vi "SEA_9811_Create_Send_Channels.vi"(8 "error in (no error)":errorcluster, 11 "Item Ref in":T1 format="%.0x") -> (0 "error out":errorcluster, 3 "Item Ref out":T1 format="%.0x")   [LabVIEW 2015, in "AIT 429 System Explorer.lvlib"]
uses:
  AIT 429 System Explorer.lvlib
  <vilib>/NI Veristand/Custom Device API/Custom Device Item Ref.ctl
  <vilib>/NI Veristand/Custom Device API/Custom Device Channel.ctl
  <vilib>/NI Veristand/Custom Device API/Custom Device Channel Type.ctl
  Shared/Controls and Global/Global.vi
  <vilib>/NI Veristand/Custom Device API/Custom Device API.lvlib
  Shared/AIT 429 Shared.lvlib
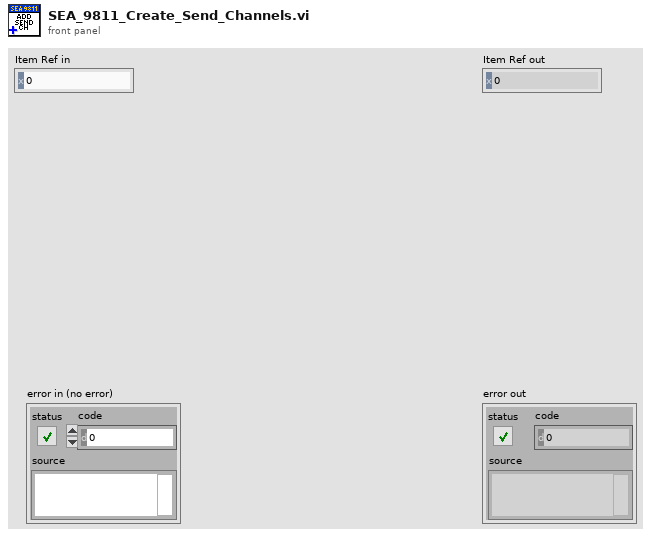
[diagram p1: front panel]
types:
  T1 = typedef "Custom Device API.lvlib/Custom Device Item Ref.ctl" = u64
  T2 = typedef "Custom Device API.lvlib/Custom Device Channel.ctl" = cluster{"Type":T3, "Units":string, "Default Value":dbl, "Faultable":bool, "Scalable":bool}
  T3 = typedef "Custom Device API.lvlib/Custom Device Channel Type.ctl" = enum16{"Input", "Output"}
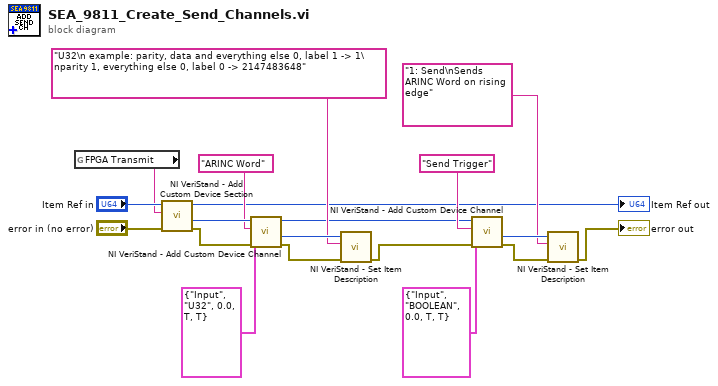
[diagram p0: block diagram]
diagram:
  n1 = global read "Global.vi" "FPGA Transmit"() -> (w1:string)
  n2 = call <vilib>:"NI VeriStand - Add Custom Device Section.vi"("error in (no error)"="error in (no error)", "Section Name"=w1, "Parent Ref in"="Item Ref in") -> ("error out"=w16:errorcluster, "Section Ptr"=w17:T1, "Parent Ref out"=→"Item Ref out":T1)  [unwired: 5 in, 1 out]
  n3 = call <vilib>:"NI VeriStand - Add Custom Device Channel.vi"("error in (no error)"=w16, "Channel"=T2 {"Type"=enum."Input", "Units"="U32", "Default Value"=0.0, "Faultable"=TRUE, "Scalable"=TRUE}, "Channel Name"="ARINC Word", "Parent Ref in"=w17) -> ("error out"=w13:errorcluster, "Channel Ref"=w12:T1, "Parent Ref out"=w8:T1)  [unwired: 4 in, 1 out]
  n4 = call <vilib>:"NI VeriStand - Set Item Description.vi"("error in (no error)"=w13, "Description"="U32\n example: parity, data and everything else 0, label 1 -> 1\nparity 1, everything else 0, label 0 -> 2147483648", "Item Ref in"=w12) -> ("error out"=w7:errorcluster)  [unwired: 6 in, 2 out]
  n5 = call <vilib>:"NI VeriStand - Add Custom Device Channel.vi"("error in (no error)"=w7, "Channel"=T2 {"Type"=enum."Input", "Units"="BOOLEAN", "Default Value"=0.0, "Faultable"=TRUE, "Scalable"=TRUE}, "Channel Name"="Send Trigger", "Parent Ref in"=w8) -> ("error out"=w5:errorcluster, "Channel Ref"=w6:T1)  [unwired: 4 in, 2 out]
  n6 = call <vilib>:"NI VeriStand - Set Item Description.vi"("error in (no error)"=w5, "Description"="1: Send\nSends ARINC Word on rising edge", "Item Ref in"=w6) -> ("error out"=→"error out":errorcluster)  [unwired: 6 in, 2 out]
